vi "Add Node To Tree.vi"(6 "Hide Passes":bool, 7 "Parent Key":string, 8 "error in (no error)":errorcluster, 9 "Test Node":T1, 10 "Key":string, 11 "tree refnum":refnum<vi>) -> (0 "error out":errorcluster, 3 "dup tree refnum":refnum<vi>)   [LabVIEW 2013, in "Caraya.lvlib" / "Basic Test Manager.lvclass"]
uses:
  Basic Test Manager.lvclass
  Test Result/Test Node.ctl
  Test Result/Test Registration Data.ctl
  Tree Symbol.ctl
  Test Result/Test Result.lvclass
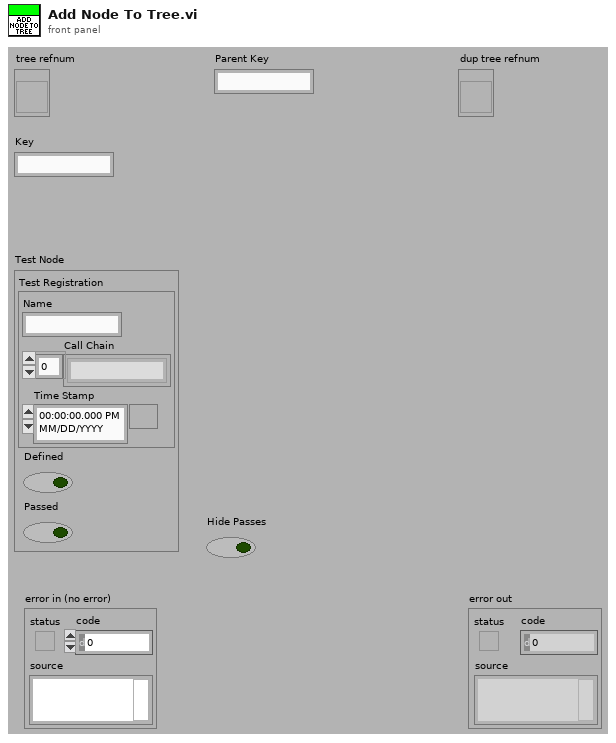
[diagram p1: front panel]
types:
  T1 = typedef "Caraya.lvlib/Test Result.lvclass/Test Node.ctl" = cluster{"Test Registration":T2, "Defined":bool, "Passed":bool}
  T2 = typedef "Caraya.lvlib/Test Result.lvclass/Test Registration Data.ctl" = cluster{"Name":string, "Call Chain":string[], "Time Stamp":timestamp}
  T3 = typedef "Caraya.lvlib/Basic Test Manager.lvclass/Tree Symbol.ctl" = enum16{"Empty", "Unknown", "Fail", "Pass", "Skip", "Error", "Fail Node", "Pass Node"}
  T4 = typedef "Caraya.lvlib/Basic Test Manager.lvclass/Test State.ctl" = enum16{"Empty", "Unknown", "Fail", "Pass", "Skip", "Error"}
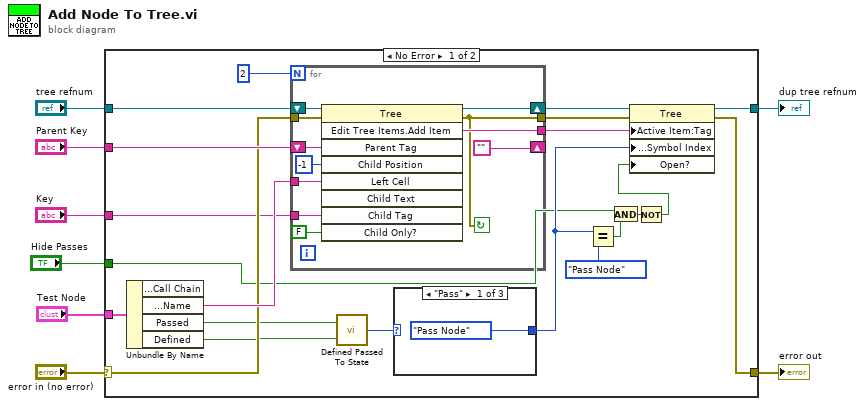
[diagram p0: block diagram]
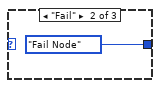
[diagram p2: hidden frame]
diagram:
  n1 = case shown="No Error" "error in (no error)" {
    selector: "error in (no error)" -> [w19 w45]
    tunnel: [w23 w45] -> w7
    tunnel: [w26 w44] -> w5
    tunnel: "tree refnum" -> [w29 w44]
    tunnel: "Parent Key" -> [w28 _]
    tunnel: "Test Node" -> [w21 _]
    tunnel: "Key" -> [w16 _]
    tunnel: "Hide Passes" -> [w11 _]
    frame No Error {
      n2 = Unbundle By Name(w21) -> ("Test Registration.Name"=w20:string, "Passed"=w18:bool, "Defined"=w17:bool)  [unwired: 1 out]
      n3 = for {
        N: 2 -> [_]
        tunnel: w20 -> [w39]
        tunnel: [w38] -> w25
        shift-right: [w40] -> w27
        shift-left: w29 -> [w43]
        tunnel: w19 -> [w37]
        tunnel: [w36] -> w24
        shift-right: [""] -> _
        shift-left: w28 -> [w42]
        tunnel: w16 -> [w33]
        stop <- w36 continue-if-true
        n4 = invoke on="Invoke Node" class="Tree" method="Edit Tree Items.Add Item"(reference=w43, error in=w37, "Parent Tag"=w42, "Child Position"=-1, "Left Cell"=w39, "Child Tag"=w33, "Child Only?"=FALSE) -> (reference out=w40:refnum<vi>, error out=w36:errorcluster, "Edit Tree Items:Add Item"=w38:string)  [unwired: 2 in, 6 out]
      }
      n5 = call "Defined Passed To State.vi"("Defined"=w17, "Passed"=w18) -> ("State"=w15:T4)
      n6 = case shown="\"Pass\"" w15 {
        selector: w15 -> [_ _ w32]
        tunnel: [Tree_Symbol."Pass Node" ("Tree Symbol") Tree_Symbol."Fail Node" ("Tree Symbol") w32] -> w14
        frame "Pass" {
        }
        frame "Fail" {
        }
        frame "Unknown", Default {
        }
      }
      n7 = Equal?(x=w14, y=Tree_Symbol."Pass Node" ("Tree Symbol")) -> (x = y?=w12:bool)
      n8 = And(x=w11, y=w12) -> (x .and. y?=w10:bool)
      n9 = Not(x=w10) -> (.not. x?=w9:bool)
      n10 = property class="Tree"(reference=w27, error in=w24, "Active Item:Tag"=w25, "Active Item:Symbol Index"=w14, "Open?"=w9) -> (reference out=w26:refnum<vi>, error out=w23:errorcluster)
    }
    frame Error {
    }
  }
  "error out" <- w7
  "dup tree refnum" <- w5
